vi "Teleop.vi"(10 "Match Info":T1={"Autonomous Elapsed Seconds"=0.0, "TeleOp Elapsed Seconds"=0.0, "Disabled Elapsed Seconds"=0.0, "Visited Autonomous"=FALSE, "Visited TeleOp"=FALSE, "Visited Disabled"=FALSE, "Autonomous Settings"={"Autonomous Style"=enum."Independent", "VI Refnum"=refnum}}, 11 "Call Context":T2) -> ()   [LabVIEW 2015]
doc: "This VI is called for each TeleOp packet received from the DS where the robot is not disabled. It is often used to read from the joysticks and update I/O or to update setpoints for timed control loops. It should complete and return within 20 milliseconds or it may miss DS packets."
uses:
  <vilib>/Rock Robotics/WPI/DriverStation/WPI_DriverStationDerivedRobotMode.ctl
  <vilib>/Rock Robotics/WPI/DriverStation/WPI_DriverStationMatch Info.ctl
  Robot Global.vi
  Robot Values.vi
  <vilib>/Rock Robotics/Network Tables/NT Read Boolean.vi
  <vilib>/Rock Robotics/Network Tables/NT Read Number.vi
  <vilib>/Rock Robotics/Network Tables/NT Write Boolean.vi
panel:
  in  "DIO out test":bool
  in  "Gyro Reset":bool
  out "Sample Slider 0":dbl(slide) scale=0.0..5.0
  out "Sample Boolean 1":bool
  out "Sample Boolean 0":bool
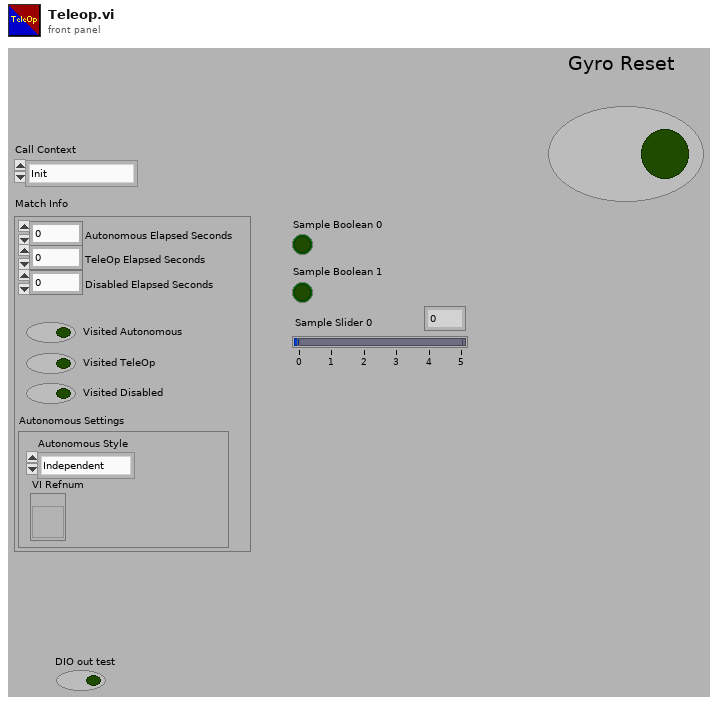
[diagram p1: front panel]
types:
  T1 = typedef "WPI_DriverStationMatch Info.ctl" = cluster{"Autonomous Elapsed Seconds":dbl, "TeleOp Elapsed Seconds":dbl, "Disabled Elapsed Seconds":dbl, "Visited Autonomous":bool, "Visited TeleOp":bool, "Visited Disabled":bool, "Autonomous Settings":cluster{"Autonomous Style":enum16{"Iterative", "Independent"}, "VI Refnum":refnum<vi>}}
  T2 = typedef "WPI_DriverStationDerivedRobotMode.ctl" = enum16{"Init", "Execute", "Stop"}
  T3 = typedef "Robot Values.ctl" = cluster{"Drive Motors":cluster{"Left Motor Value":dbl, "Right Motor Value":dbl, "Left Motor Encoder":dbl, "Right Motor Encoder":dbl, "High/Low Gear":bool}, "Sensors":cluster{"Gyro Angle":dbl, "Photoeye":bool, "Ultrasonic Range":dbl, "Shooter Speed Encoder":dbl, "Accelerometer Value":dbl, "Flashlight":bool, "Target Distance":dbl, "Target X Value":dbl, "Reset Gyro?":bool}, "Arms":cluster{"Desired Arm Position":dbl, "Left Arm Encoder":dbl, "Right Arm Encoder":dbl, "Left Arm Lower Limit":bool, "Right Arm Lower Limit":bool, "Initialize Arm Position?":bool}, "Acquisition and Scoring":cluster{"Acquiring?":bool, "Current Speed":dbl, "Setpoint Speed":dbl, "Prep Wheels":bool, "Shoot":bool, "Low Eject":bool, "Reverse Shooter Wheel":bool}, "Hanging":cluster{"Pivot Arms":dbl, "PTO":bool, "Left Pivot Encoder":dbl, "Right Pivot Encoder":dbl, "Hanging Pin":bool}}
  T4 = typedef "Robot Drive.ctl" = cluster{"RobotDriveDevRef":T5, "Joysticks":cluster{"JoystickDevRef":T13, "JoystickDevRef 2":T13}, "Sensor":T15, "Pneumatics":T34, "Defenses":cluster{"LeftArm MotorControlDeviceRef":T6, "RightArm MotorControlDeviceRef":T6}, "Hanging":cluster{"Left Erection MotorControlDeviceRef":T6, "Right Erection MotorControlDeviceRef":T6}, "Aquisition + Scoring":T38, "DigitalOutputDevRef":T42, "DigitalInputDevRef":T19}
  T5 = typedef "WPI_RobotDriveDevRef.ctl" = cluster{"DevStatus":errorcluster, "Motors[]":T6[], "Square Inputs":bool, "Max Output":dbl}
  T6 = typedef "WPI_MotorControlDeviceRef.ctl" = cluster{"DeviceStatus":errorcluster, "Type":T7, "PWM":cluster{"PWM Channel":T8, "DeadBand":T9}, "CAN":cluster{"Device Number":u8, "Control Mode":T10, "Semaphore":T11, "Max Vout":dbl, "TalonSRX Control Mode":T12}, "Invert":bool}
  T7 = typedef "WPI_MotorControlType.ctl" = enum16{"PWM", "CAN", "CANTalonSRX"}
  T8 = typedef "FPGA_DIOPWMChannel.ctl" = enum8{"PWM 0", "PWM 1", "PWM 2", "PWM 3", "PWM 4", "PWM 5", "PWM 6", "PWM 7", "PWM 8", "PWM 9", "PWM MXP 0", "PWM MXP 1", "PWM MXP 2", "PWM MXP 3", "PWM MXP 4", "PWM MXP 5", "PWM MXP 6", "PWM MXP 7", "PWM MXP 8", "PWM MXP 9", "Invalid"}
  T9 = typedef "WPI_PWMDeadband.ctl" = cluster{"Name":string, "maxPositivePwm":i32, "minPositivePwm":i32, "centerPwm":i32, "maxNegativePwm":i32, "minNegativePwm":i32, "angularRange":u16}
  T10 = typedef "WPI_CANJaguar_ControlMode.ctl" = enum8{"Percent VBus", "Current", "Speed", "Position", "Voltage"}
  T11 = typedef "Semaphore RefNum" = refnum<k1>
  T12 = typedef "WPI_CANTalonSRX_APIControlMode.ctl" = enum8{"Percent VBus", "Speed", "Position", "Slave", "Unchanged / Invalid", "Voltage Compensation", "Current", "Motion Profile"}
  T13 = typedef "WPI_JoystickDevRef.ctl" = cluster{"Device":T14}
  T14 = typedef "WPI_JoystickDeviceEnum.ctl" = enum16{"USB 0", "USB 1", "USB 2", "USB 3", "USB 4", "USB 5"}
  T15 = typedef "Sensors.ctl" = cluster{"GyroDevRef":T16, "Left Arm Limit DigitalInputDevRef":T19, "Right Arm Limit DigitalInputDevRef":T19, "Left Arm EncoderDevRef":T21, "Right Arm EncoderDevRef":T21, "Left Drive EncoderDevRef":T21, "Right Drive EncoderDevRef":T21, "BoB Photoeye DigitalInputDevRef":T19, "Range SonarMB1010AnalogDevRef":T25, "Shooter CounterDevRef":T27, "AccelerometerDevRef":T28, "Left Hanging Erecter EncoderDevRef":T21, "Right Hanging Erecter EncoderDevRef":T21, "TestDigitalInputDevRef":T19}
  T16 = typedef "WPI_GyroDevRef.ctl" = cluster{"DevStatus":errorcluster, "Analog Channel":T17, "Offset":dbl, "Gain (VoltsPerDegree/Second)":dbl, "Gyro Type":enum16{"Analog", "XRS450"}, "Handle":i32, "SPI Bus":T18, "Device Found":bool, "Sample Rate":dbl, "Calibrate On Open":bool}
  T17 = typedef "FPGA_AIChannel.ctl" = enum8{"AI 0", "AI 1", "AI 2", "AI 3", "AI MXP 0", "AI MXP 1", "AI MXP 2", "AI MXP 3", "Invalid"}
  T18 = typedef "spi_bus.ctl" = enum16{"SPI On-Board, CS0", "SPI On-Board, CS1", "SPI On-Board, CS2", "SPI On-Board, CS3", "SPI MXP", "Invalid"}
  T19 = typedef "WPI_DigitalInputDevRef.ctl" = cluster{"DevStatus":errorcluster, "DIO Channel":T20}
  T20 = typedef "FPGA_DIOChannel.ctl" = enum8{"DIO 0", "DIO 1", "DIO 2", "DIO 3", "DIO 4", "DIO 5", "DIO 6", "DIO 7", "DIO 8", "DIO 9", "DIO MXP 0", "DIO MXP 1", "DIO MXP 2", "DIO MXP 3", "DIO MXP 4", "DIO MXP 5", "DIO MXP 6", "DIO MXP 7", "DIO MXP 8", "DIO MXP 9", "DIO MXP 10", "DIO MXP 11", "DIO MXP 12", "DIO MXP 13", "DIO MXP 14", "DIO MXP 15", "Invalid"}
  T21 = typedef "WPI_EncoderDevRef.ctl" = cluster{"DevStatus":errorcluster, "EncoderIndex":T22, "CounterIndex":T23, "DistancePerCount":dbl, "Decoding Type":T24}
  T22 = typedef "FPGA_EncoderIdx.ctl" = enum8{"Enc 0", "Enc 1", "Enc 2", "Enc 3", "Enc 4", "Enc 5", "Enc 6", "Enc 7", "Invalid"}
  T23 = typedef "FPGA_CounterCtrSystemIndex.ctl" = enum8{"Ctr 0", "Ctr 1", "Ctr 2", "Ctr 3", "Ctr 4", "Ctr 5", "Ctr 6", "Ctr 7", "Invalid"}
  T24 = typedef "WPI_EncoderType.ctl" = enum16{"1x", "2x", "4x"}
  T25 = typedef "WPI_SonarMB1010AnalogDeviceRef.ctl" = cluster{"AIDeviceRef":T26, "Scaling factor (V/in)":dbl, "Average Bits":u8}
  T26 = typedef "WPI_AnalogChannelDevRef.ctl" = cluster{"DevStatus":errorcluster, "Analog Channel":T17}
  T27 = typedef "WPI_CounterDevRef.ctl" = cluster{"DevStatus":errorcluster, "CntIndex":T23}
  T28 = typedef "WPI_AccelerometerDevRef.ctl" = cluster{"DevStatus":errorcluster, "Scaling":T29, "Analog Channels":T30, "I2C Bus":T31, "SPI Bus":T18, "Accel Range":T32, "ADXL Axes":T33, "Handle":i32, "Device Address":u8, "Accel Type":enum16{"Analog", "ADXL345 I2C", "ADXL345 SPI", "Internal", "ADXL362 SPI"}}
  T29 = typedef "WPI_AccelerometerScaling.ctl" = cluster{"Gain (VoltsPerG)":dbl, "Center Voltage":dbl}
  T30 = typedef "WPI_AccelerometerAnalogChannels.ctl" = cluster{"X-Axis":T17, "Y-Axis":T17, "Z-Axis":T17}
  T31 = typedef "i2c_bus.ctl" = enum16{"I2C On-Board", "I2C MXP", "Invalid"}
  T32 = typedef "ADXL345 Range.ctl" = u8
  T33 = typedef "WPI_AccelerometerADXL345 Axes.ctl" = cluster{"X-Axis":bool, "Y-Axis":bool, "Z-Axis":bool}
  T34 = typedef "Pnematics.ctl" = cluster{"CompressorDevRef":T35, "High and Low Gear DoubleSolenoidDevRef":T36, "PTO SolenoidDevRef":T36, "Hang Pin SolenoidDevRef":T36}
  T35 = typedef "WPI_CompressorDevRef.ctl" = cluster{"DevStatus":errorcluster, "Pneumatics Control Module":u8}
  T36 = typedef "WPI_SolenoidDevRef.ctl" = cluster{"DevStatus":errorcluster, "Pneumatics Control Module":u8, "Forward Solenoid Channel":T37, "Reverse Solenoid Channel":T37}
  T37 = typedef "WPI_SolenoidChannel.ctl" = enum8{"Solenoid 0", "Solenoid 1", "Solenoid 2", "Solenoid 3", "Solenoid 4", "Solenoid 5", "Solenoid 6", "Solenoid 7", "Invalid"}
  T38 = typedef "Acquisition & Scoring.ctl" = cluster{"Outer Roller MotorControlDeviceRef":T6, "Inner Roller MotorControlDeviceRef":T6, "Scoring Top MotorControlDeviceRef":T6, "Scoring Bottom MotorControlDeviceRef":T6, "Flashlight RelayDevRef":T39}
  T39 = typedef "WPI_RelayDevRef.ctl" = cluster{"DevStatus":errorcluster, "Relay Channel":T40, "Relay Direction":T41}
  T40 = typedef "FPGA_DIORelayChannel.ctl" = enum8{"Relay 0", "Relay 1", "Relay 2", "Relay 3", "Invalid"}
  T41 = typedef "WPI_RelayDirection.ctl" = enum16{"Both directions", "Forward only", "Reverse only"}
  T42 = typedef "WPI_DigitalOutputDevRef.ctl" = cluster{"DIO Channel":T20, "DevStatus":errorcluster}
  T43 = cluster{"Left":dbl, "Right":dbl, "Gear":bool, "PTO":bool, "Rear Camera":bool, "Hanging Pin":bool}
  T44 = cluster{"Position out":dbl, "Acquiring":bool, "Shoot":bool, "Prep Wheels":bool, "Low Eject":bool, "Pivot Hooks":dbl, "Reverse Shooter Wheel":bool}
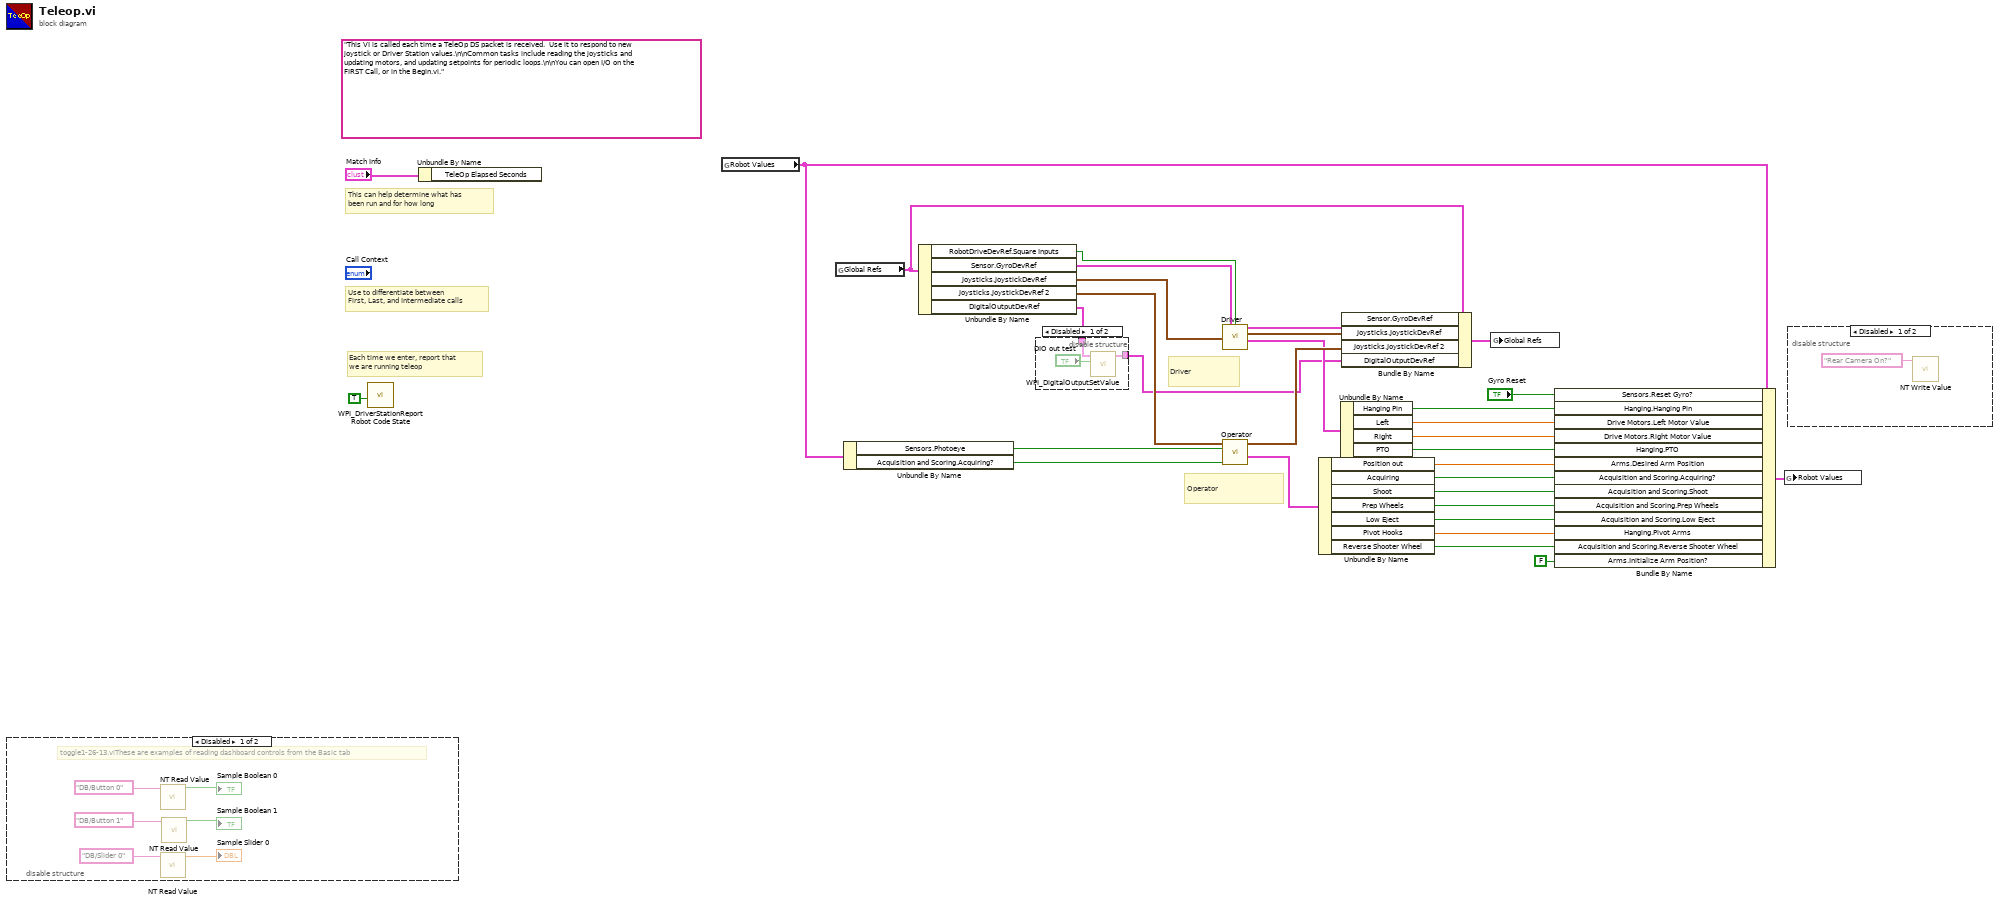
[diagram p0: block diagram]
diagram:
  (unwired) "This VI is called each time a TeleOp DS packet is received.  Use it to respond to new joystick or Driver Station values.\n\nCommon tasks include reading the joysticks and updating motors, and updating setpoints for periodic loops.\n\nYou can open I/O on the FIRST Call, or in the Begin.vi."
  # "Driver"
  # "Operator"
  # "Each time we enter, report that\nwe are running teleop"
  # "Use to differentiate between\nFirst, Last, and Intermediate calls"
  # "This can help determine what has\nbeen run and for how long"
  n1 = disable-structure shown="Disabled" {
    frame Disabled {
      # "toggle1-26-13.viThese are examples of reading dashboard controls from the Basic tab"
      n2 = call-poly <vilib>:"NT Read Value.vi"("Name"="DB/Button 0" ("refnum name")) -> ("Boolean"=→"Sample Boolean 0":bool)  [unwired: 9 in, 1 out]
      n3 = call-poly <vilib>:"NT Read Value.vi"("Name"="DB/Slider 0" ("refnum name")) -> ("Numeric"=→"Sample Slider 0":dbl)  [unwired: 9 in, 1 out]
      n4 = call-poly <vilib>:"NT Read Value.vi"("Name"="DB/Button 1" ("refnum name")) -> ("Boolean"=→"Sample Boolean 1":bool)  [unwired: 9 in, 1 out]
    }
    frame Enabled {
    }
  }
  n5 = call <vilib>:"WPI_DriverStationReport Robot Code State.vi"("TeleOp"=TRUE ("Autonomous")) -> ()  [unwired: 10 in, 1 out]
  n6 = Unbundle By Name("Match Info") -> ()  [unwired: 1 out]
  n7 = global read "Robot Values.vi" "Robot Values"() -> (w10:T3)
  n8 = global read "Robot Global.vi" "Global Refs"() -> (w22:T4)
  n9 = Unbundle By Name(w10) -> ("Sensors.Photoeye"=w9:bool, "Acquisition and Scoring.Acquiring?"=w8:bool)
  n10 = Unbundle By Name(w22) -> ("RobotDriveDevRef.Square Inputs"=w25:bool, "Sensor.GyroDevRef"=w27:T16, "Joysticks.JoystickDevRef"=w30:T13, "Joysticks.JoystickDevRef 2"=w24:T13, "DigitalOutputDevRef"=w5:T42)
  n11 = disable-structure shown="Disabled" {
    disable-tunnel: w5 -> [w41 _]
    disable-tunnel: [w40 _] -> w4
    frame Disabled {
      n12 = call <vilib>:"WPI_DigitalOutputSetValue.vi"("Value"="DIO out test", "DigitalOutputDevRef"=w41) -> ("DigitalOutputDevRef"=w40:T42)  [unwired: 8 in, 1 out]
    }
    frame Enabled {
    }
  }
  n13 = call "Driver.vi"("GyroDevRef in"=w27, "Square Inputs"=w25, "JoystickDevRef in"=w30) -> ("GyroDevRef out"=w28:T16, "JoystickDevRef out"=w26:T13, "Output"=w14:T43)  [unwired: 10 in]
  n14 = call "Operator.vi"("Aquiring?"=w8, "Photoeye"=w9, "JoystickDevRef in"=w24) -> ("Output"=w20:T44, "JoystickDevRef out"=w23:T13)  [unwired: 7 in]
  n15 = Unbundle By Name(w20) -> ("Position out"=w19:dbl, "Acquiring"=w18:bool, "Shoot"=w17:bool, "Prep Wheels"=w16:bool, "Low Eject"=w15:bool, "Pivot Hooks"=w7:dbl, "Reverse Shooter Wheel"=w2:bool)
  n16 = Unbundle By Name(w14) -> ("Hanging Pin"=w6:bool, "Left"=w12:dbl, "Right"=w11:dbl, "PTO"=w13:bool)
  n17 = Bundle By Name(cluster=w22, "Sensor.GyroDevRef"=w28, "Joysticks.JoystickDevRef"=w26, "Joysticks.JoystickDevRef 2"=w23, "DigitalOutputDevRef"=w4) -> (w29:T4)
  n18 = global write "Robot Global.vi" "Global Refs"(w29) -> ()
  n19 = Bundle By Name(cluster=w10, "Sensors.Reset Gyro?"="Gyro Reset", "Hanging.Hanging Pin"=w6, "Drive Motors.Left Motor Value"=w12, "Drive Motors.Right Motor Value"=w11, "Hanging.PTO"=w13, "Arms.Desired Arm Position"=w19, "Acquisition and Scoring.Acquiring?"=w18, "Acquisition and Scoring.Shoot"=w17, "Acquisition and Scoring.Prep Wheels"=w16, "Acquisition and Scoring.Low Eject"=w15, "Hanging.Pivot Arms"=w7, "Acquisition and Scoring.Reverse Shooter Wheel"=w2, "Arms.Initialize Arm Position?"=FALSE) -> (w21:T3)
  n20 = global write "Robot Values.vi" "Robot Values"(w21) -> ()
  n21 = disable-structure shown="Disabled" {
    frame Disabled {
      n22 = call-poly <vilib>:"NT Write Value.vi"("Name"="Rear Camera On?") -> ()  [unwired: 10 in, 1 out]
    }
    frame Enabled {
    }
  }
